vi "Sort Contacts.vi"(8 "error in (no error)":errorcluster, 9 "Ascending? (T)":bool=TRUE, 10 "Sort Mode (Default)":T1 items=["Default", "Last Name", "First Name", "Middle Name", "Phone", "Street", "City", "State", "Postal Code", "Favorite"], 11 "Contacts":T2[](array[typedef])) -> (0 "error out":errorcluster, 3 "Sorted Contacts":T2[](array[typedef]))   [LabVIEW 2014, in "Contact Data.lvlib"]
doc: "Sorts an array of contacts based on a sort mode and order."
uses:
  Contact Data.lvlib
  Position.ctl
  Contact.ctl
  Control Sort Mode.ctl
  Controls.ctl
  DesinationControls.ctl
  DestinationCluster.ctl
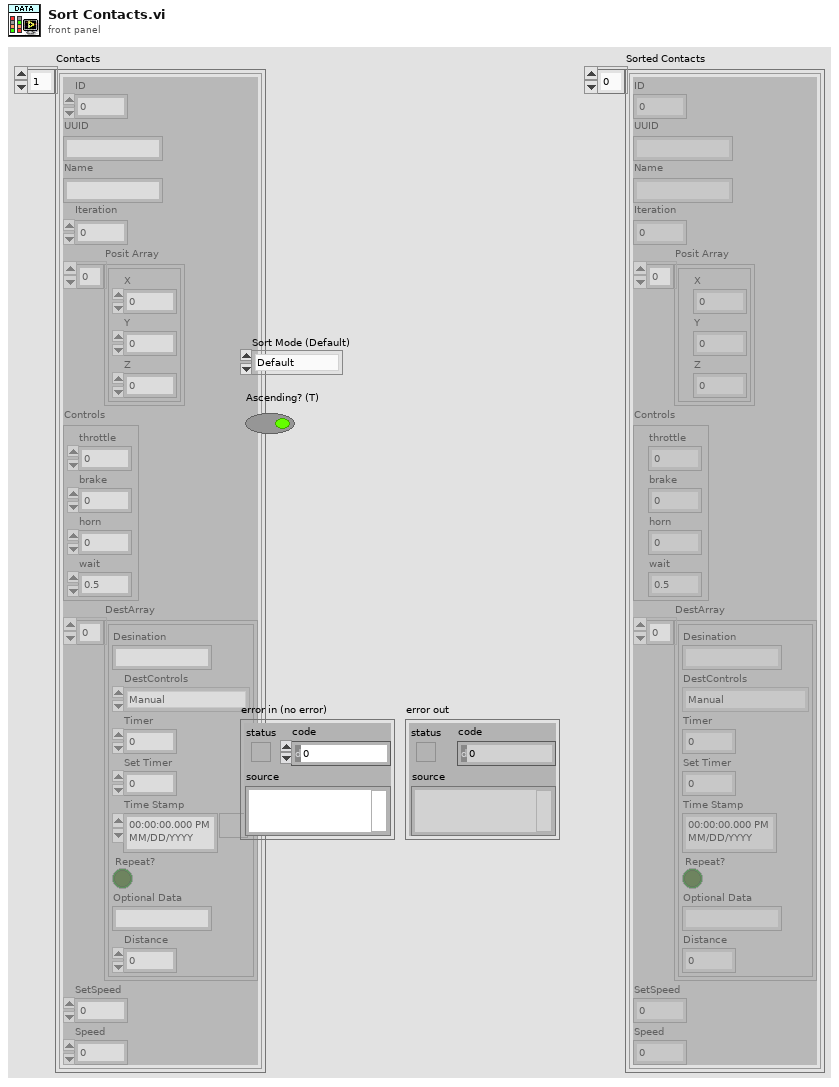
[diagram p1: front panel]
types:
  T1 = typedef "Contact Data.lvlib/Control Sort Mode.ctl" = u16
  T2 = typedef "Contact Data.lvlib/Contact.ctl" = cluster{"ID":u32, "UUID":string, "Name":string, "Iteration":i32, "Posit Array":T3[], "Controls":T4, "DestArray":T5[], "SetSpeed":dbl, "Speed":dbl}
  T3 = typedef "Contact Data.lvlib/Position.ctl" = cluster{"X":dbl, "Y":dbl, "Z":dbl}
  T4 = typedef "Contact Data.lvlib/Controls.ctl" = cluster{"throttle":dbl, "brake":dbl, "horn":dbl, "wait":dbl}
  T5 = typedef "Contact Data.lvlib/DestinationCluster.ctl" = cluster{"Desination":string, "DestControls":T6, "Timer":u32, "Set Timer":u32, "Time Stamp":timestamp, "Repeat?":bool, "Optional Data":string, "Distance":dbl}
  T6 = typedef "Contact Data.lvlib/DesinationControls.ctl" = enum16{"Tracker", "Manual", "Stop", "Station DateTime", "Station Timer", "Maintain"}
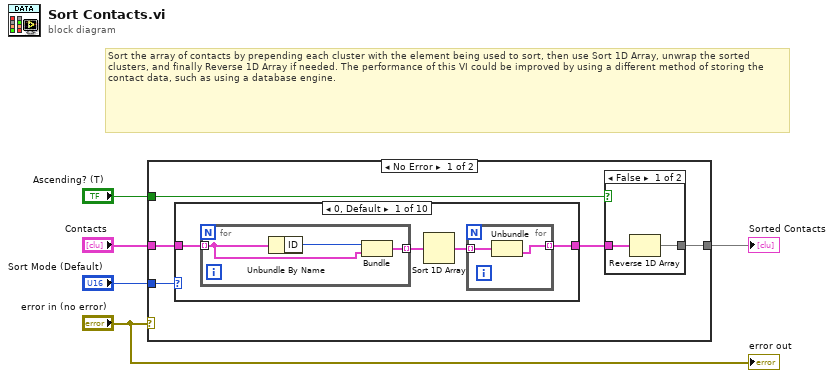
[diagram p0: block diagram]
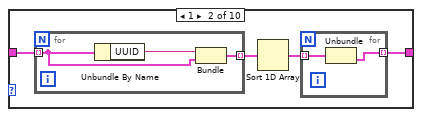
[diagram p2: hidden frame]
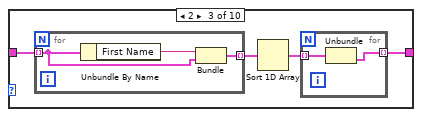
[diagram p3: hidden frame]
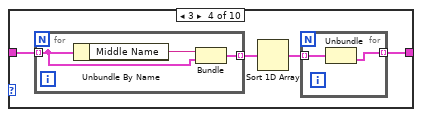
[diagram p4: hidden frame]
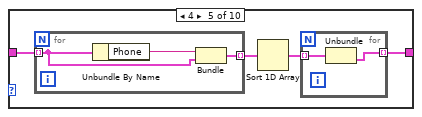
[diagram p5: hidden frame]
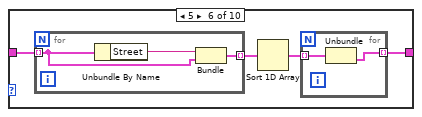
[diagram p6: hidden frame]
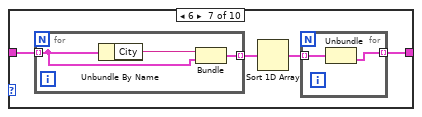
[diagram p7: hidden frame]
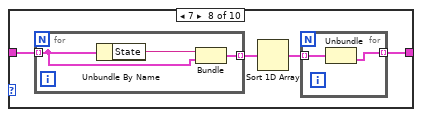
[diagram p8: hidden frame]
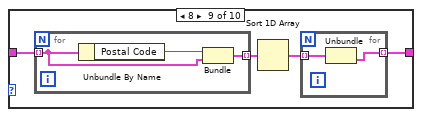
[diagram p9: hidden frame]
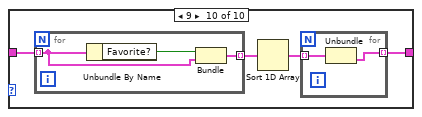
[diagram p10: hidden frame]
diagram:
  # "Sort the array of contacts by prepending each cluster with the element being used to sort, then use Sort 1D Array, unwrap the sorted clusters, and finally Reverse 1D Array if needed. The performance of this VI could be improved by using a different method of storing the contact data, such as using a database engine."
  n1 = case shown="No Error" "error in (no error)" {
    tunnel: "Ascending? (T)" -> [w7 _]
    tunnel: "Contacts" -> [w8 w104]
    tunnel: [w10 w104] -> w3
    tunnel: "Sort Mode (Default)" -> [w9 _]
    frame No Error {
      n2 = case shown="0, Default" w9 {
        tunnel: w8 -> [w14 w23 w32 w41 w50 w59 w68 w77 w86 w95]
        tunnel: [w11 w20 w29 w38 w47 w56 w65 w74 w83 w92] -> w6
        frame 0, Default {
          n3 = for {
            tunnel: w14 -> [w18] mode=indexing
            tunnel: [w17] -> w13 mode=indexing
            n4 = Unbundle By Name(w18) -> ("ID"=w19:u32)
            n5 = Bundle("ID"=w19, "Contact"=w18) -> (w17:cluster{"ID":u32, "Contact":T2})  [unwired: 1 in]
          }
          n6 = Sort 1D Array(array=w13) -> (sorted array=w12:cluster{"ID":u32, "Contact":T2}[])
          n7 = for {
            tunnel: w12 -> [w16] mode=indexing
            tunnel: [w15] -> w11 mode=indexing
            n8 = Unbundle(w16) -> ("Contact"=w15:T2)  [unwired: 1 out]
          }
        }
        frame 1 {
          n9 = for {
            tunnel: w23 -> [w27] mode=indexing
            tunnel: [w26] -> w22 mode=indexing
            n10 = Unbundle By Name(w27) -> ("UUID"=w28:string)
            n11 = Bundle("UUID"=w28, "Contact"=w27) -> (w26:cluster{"UUID":string, "Contact":T2})  [unwired: 1 in]
          }
          n12 = Sort 1D Array(array=w22) -> (sorted array=w21:cluster{"UUID":string, "Contact":T2}[])
          n13 = for {
            tunnel: w21 -> [w25] mode=indexing
            tunnel: [w24] -> w20 mode=indexing
            n14 = Unbundle(w25) -> ("Contact"=w24:T2)  [unwired: 1 out]
          }
        }
        frame 2 {
          n15 = for {
            tunnel: w32 -> [w36] mode=indexing
            tunnel: [w35] -> w31 mode=indexing
            n16 = Unbundle By Name(w36) -> ("First Name"=w37:string)
            n17 = Bundle("First Name"=w37, "Contact"=w36) -> (w35:cluster{"First Name":string, "Contact":T2})  [unwired: 1 in]
          }
          n18 = Sort 1D Array(array=w31) -> (sorted array=w30:cluster{"First Name":string, "Contact":T2}[])
          n19 = for {
            tunnel: w30 -> [w34] mode=indexing
            tunnel: [w33] -> w29 mode=indexing
            n20 = Unbundle(w34) -> ("Contact"=w33:T2)  [unwired: 1 out]
          }
        }
        frame 3 {
          n21 = for {
            tunnel: w41 -> [w45] mode=indexing
            tunnel: [w44] -> w40 mode=indexing
            n22 = Unbundle By Name(w45) -> ("Middle Name"=w46:string)
            n23 = Bundle("Middle Name"=w46, "Contact"=w45) -> (w44:cluster{"Middle Name":string, "Contact":T2})  [unwired: 1 in]
          }
          n24 = Sort 1D Array(array=w40) -> (sorted array=w39:cluster{"Middle Name":string, "Contact":T2}[])
          n25 = for {
            tunnel: w39 -> [w43] mode=indexing
            tunnel: [w42] -> w38 mode=indexing
            n26 = Unbundle(w43) -> ("Contact"=w42:T2)  [unwired: 1 out]
          }
        }
        frame 4 {
          n27 = for {
            tunnel: w50 -> [w54] mode=indexing
            tunnel: [w53] -> w49 mode=indexing
            n28 = Unbundle By Name(w54) -> ("Phone"=w55:string)
            n29 = Bundle("Phone"=w55, "Contact"=w54) -> (w53:cluster{"Phone":string, "Contact":T2})  [unwired: 1 in]
          }
          n30 = Sort 1D Array(array=w49) -> (sorted array=w48:cluster{"Phone":string, "Contact":T2}[])
          n31 = for {
            tunnel: w48 -> [w52] mode=indexing
            tunnel: [w51] -> w47 mode=indexing
            n32 = Unbundle(w52) -> ("Contact"=w51:T2)  [unwired: 1 out]
          }
        }
        frame 5 {
          n33 = for {
            tunnel: w59 -> [w63] mode=indexing
            tunnel: [w62] -> w58 mode=indexing
            n34 = Unbundle By Name(w63) -> ("Street"=w64:string)
            n35 = Bundle("Street"=w64, "Contact"=w63) -> (w62:cluster{"Street":string, "Contact":T2})  [unwired: 1 in]
          }
          n36 = Sort 1D Array(array=w58) -> (sorted array=w57:cluster{"Street":string, "Contact":T2}[])
          n37 = for {
            tunnel: w57 -> [w61] mode=indexing
            tunnel: [w60] -> w56 mode=indexing
            n38 = Unbundle(w61) -> ("Contact"=w60:T2)  [unwired: 1 out]
          }
        }
        frame 6 {
          n39 = for {
            tunnel: w68 -> [w72] mode=indexing
            tunnel: [w71] -> w67 mode=indexing
            n40 = Unbundle By Name(w72) -> ("City"=w73:string)
            n41 = Bundle("City"=w73, "Contact"=w72) -> (w71:cluster{"City":string, "Contact":T2})  [unwired: 1 in]
          }
          n42 = Sort 1D Array(array=w67) -> (sorted array=w66:cluster{"City":string, "Contact":T2}[])
          n43 = for {
            tunnel: w66 -> [w70] mode=indexing
            tunnel: [w69] -> w65 mode=indexing
            n44 = Unbundle(w70) -> ("Contact"=w69:T2)  [unwired: 1 out]
          }
        }
        frame 7 {
          n45 = for {
            tunnel: w77 -> [w81] mode=indexing
            tunnel: [w80] -> w76 mode=indexing
            n46 = Unbundle By Name(w81) -> ("State"=w82:string)
            n47 = Bundle("State"=w82, "Contact"=w81) -> (w80:cluster{"State":string, "Contact":T2})  [unwired: 1 in]
          }
          n48 = Sort 1D Array(array=w76) -> (sorted array=w75:cluster{"State":string, "Contact":T2}[])
          n49 = for {
            tunnel: w75 -> [w79] mode=indexing
            tunnel: [w78] -> w74 mode=indexing
            n50 = Unbundle(w79) -> ("Contact"=w78:T2)  [unwired: 1 out]
          }
        }
        frame 8 {
          n51 = for {
            tunnel: w86 -> [w90] mode=indexing
            tunnel: [w89] -> w85 mode=indexing
            n52 = Unbundle By Name(w90) -> ("Postal Code"=w91:string)
            n53 = Bundle("Postal Code"=w91, "Contact"=w90) -> (w89:cluster{"Postal Code":string, "Contact":T2})  [unwired: 1 in]
          }
          n54 = Sort 1D Array(array=w85) -> (sorted array=w84:cluster{"Postal Code":string, "Contact":T2}[])
          n55 = for {
            tunnel: w84 -> [w88] mode=indexing
            tunnel: [w87] -> w83 mode=indexing
            n56 = Unbundle(w88) -> ("Contact"=w87:T2)  [unwired: 1 out]
          }
        }
        frame 9 {
          n57 = for {
            tunnel: w95 -> [w99] mode=indexing
            tunnel: [w98] -> w94 mode=indexing
            n58 = Unbundle By Name(w99) -> ("Favorite?"=w100:bool)
            n59 = Bundle("Favorite?"=w100, "Contact"=w99) -> (w98:cluster{"Favorite?":bool, "Contact":T2})  [unwired: 1 in]
          }
          n60 = Sort 1D Array(array=w94) -> (sorted array=w93:cluster{"Favorite?":bool, "Contact":T2}[])
          n61 = for {
            tunnel: w93 -> [w97] mode=indexing
            tunnel: [w96] -> w92 mode=indexing
            n62 = Unbundle(w97) -> ("Contact"=w96:T2)  [unwired: 1 out]
          }
        }
      }
      n63 = case shown="False" w7 {
        tunnel: w6 -> [w102 w103]
        tunnel: [w101 w103] -> w10
        frame False {
          n64 = Reverse 1D Array(array=w102) -> (reversed array=w101:T2[])
        }
        frame True {
        }
      }
    }
    frame Error {
    }
  }
  "Sorted Contacts" <- w3
  "error out" <- "error in (no error)"
